vi "Measure High and Low States.vi"(8 "error in":errorcluster, 11 "signal in":waveform(dbl)) -> (0 "error out":errorcluster, 2 "final state level":dbl, 3 "inital state level":dbl)   [LabVIEW 2010]
uses:
  <vilib>/measure/mascope.llb/Amplitude and Levels 1 chan.vi
  <vilib>/measure/mamon.llb/Trigger Detection for 1 Channel.vi
  <vilib>/measure/NI_MAPro.lvlib
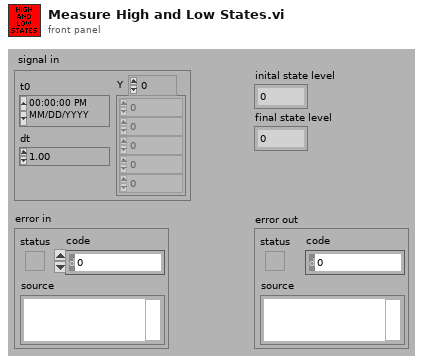
[diagram p1: front panel]
types:
  T1 = cluster{"method":enum32{"histogram", "peak", "auto select"}, "histogram size":i32, "histogram method":enum16{"mode"}, "reserved":dbl}
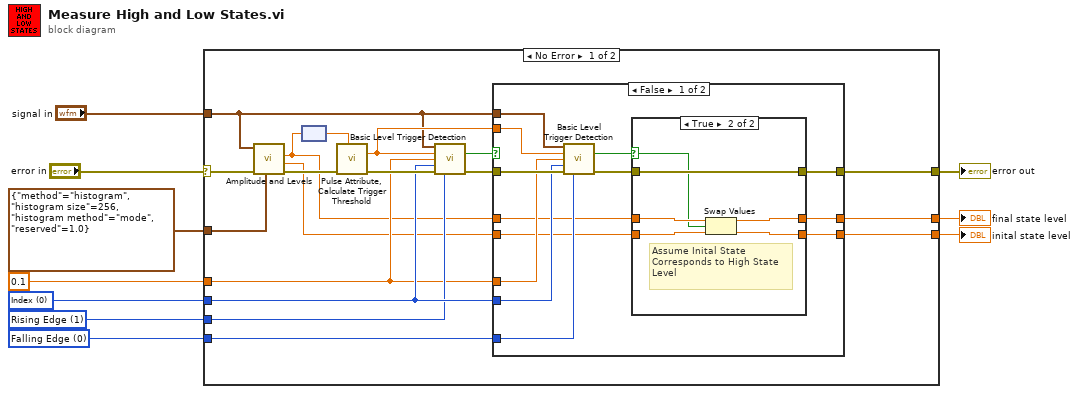
[diagram p0: block diagram]
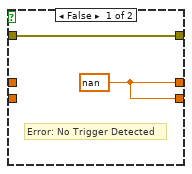
[diagram p2: hidden frame]
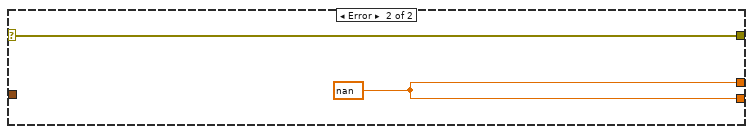
[diagram p4: hidden frame]
diagram:
  w7 = u16 0 items=["Falling Edge", "Rising Edge"] ("trigger slope")
  w9 = u16 0 items=["Index", "Time"] ("location mode")
  w8 = u16 1 items=["Falling Edge", "Rising Edge"] ("trigger slope")
  n1 = case shown="No Error" "error in" {
    selector: "error in" -> [w16 w54]
    tunnel: T1 {"method"=enum."histogram", "histogram size"=256, "histogram method"=enum."mode", "reserved"=1.0} ("state settings") -> [w28 _]
    tunnel: w9 -> [w21 _]
    tunnel: w8 -> [w20 _]
    tunnel: w7 -> [w19 _]
    tunnel: "signal in" -> [w18 _]
    tunnel: 0.1 ("hysteresis") -> [w17 _]
    tunnel: [w13 w53] -> w3
    tunnel: [w12 w53] -> w2
    tunnel: [w11 w54] -> w1
    frame No Error {
      n2 = call-poly <vilib>:"Amplitude and Levels.vi"("state settings"=w28, "error in (no error)"=w16, "signal in"=w18) -> ("error out"=w26:errorcluster, "low state level"=w15:dbl, "high state level"=w14:dbl)  [unwired: 5 in, 1 out]
      n3 = node(w14) -> (w24:dbl[unit])
      n4 = call "Pulse Attribute, Calculate Trigger Threshold.vi"("pulse amp"=w24, "error in"=w26) -> ("error out"=w25:errorcluster, "trigger level (V)"=w22:dbl)  [unwired: 5 in]
      n5 = call-poly <vilib>:"Basic Level Trigger Detection.vi"("signal in"=w18, "level"=w22, "hysteresis"=w17, "location mode"=w21, "error in (no error)"=w25, "trigger slope"=w20) -> ("trigger detected?"=w27:bool, "error out"=w23:errorcluster)  [unwired: 7 in, 1 out]
      n6 = case shown="False" w27 {
        tunnel: w23 -> [w41 w50]
        tunnel: w22 -> [w40 _]
        tunnel: w21 -> [w39 _]
        tunnel: w19 -> [w38 _]
        tunnel: w18 -> [w37 _]
        tunnel: w17 -> [w36 _]
        tunnel: w15 -> [w31 w51]
        tunnel: w14 -> [w32 w52]
        tunnel: [w30 w52] -> w13
        tunnel: [w29 w51] -> w12
        tunnel: [w33 w50] -> w11
        frame False {
          n7 = call-poly <vilib>:"Basic Level Trigger Detection.vi"("signal in"=w37, "level"=w40, "hysteresis"=w36, "location mode"=w39, "error in (no error)"=w41, "trigger slope"=w38) -> ("trigger detected?"=w35:bool, "error out"=w34:errorcluster)  [unwired: 7 in, 1 out]
          n8 = case shown="True" w35 {
            selector: w35 -> [_ w44]
            tunnel: w34 -> [w42 w49]
            tunnel: [w42 w49] -> w33
            tunnel: w32 -> [_ w48]
            tunnel: w31 -> [_ w47]
            tunnel: [w43 w46] -> w30
            tunnel: [w43 w45] -> w29
            frame False {
              w43 = nan
              # "Error: No Trigger Detected"
            }
            frame True {
              # "Assume Inital State\t\nCorresponds to High State\nLevel"
              n9 = Swap Values(12:w48, 13:w44, 14:w47) -> (1:w46:dbl, 3:w45:dbl)
            }
          }
        }
        frame True {
          # "Assume \"Inital State\" corresponds to the \"Low State Level\""
        }
      }
    }
    frame Error {
      w53 = nan
    }
  }
  "final state level" <- w3
  "inital state level" <- w2
  "error out" <- w1
